vi "Write Response OK.vi"(0 "connection ID":refnum<k5>, 7 "Payload":string="{}", 9 "timeout (ms)":i32=5000, 11 "error in (no error)":errorcluster) -> (4 "connection ID out":refnum<k5>, 15 "error out":errorcluster)   [LabVIEW 2020, in "epl-network.lvlib"]
uses:
  epl-network.lvlib
  Typedefs/TCP Message.ctl
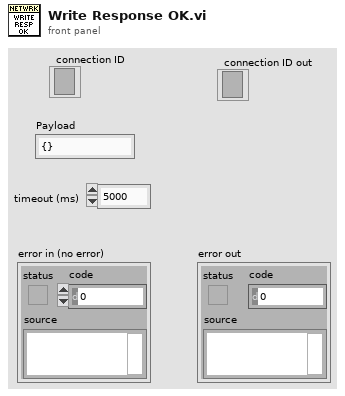
[diagram p1: front panel]
types:
  T1 = typedef "epl-network.lvlib/TCP Message.ctl" = cluster{"Code":i32, "Command":string, "Payload":string}
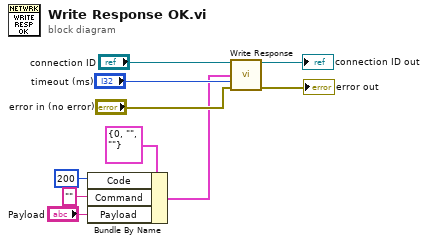
[diagram p0: block diagram]
diagram:
  n1 = Bundle By Name(cluster=T1 {"Code"=0, "Command"="", "Payload"=""} ("TCPMessage"), "Code"=200, "Command"="", "Payload"="Payload") -> (w3:T1)
  n2 = call "Write Response.vi"("connection ID"="connection ID", "TCPMessage"=w3, "timeout (ms)"="timeout (ms)", "error in (no error)"="error in (no error)") -> ("connection ID out"=→"connection ID out":refnum<k5>, "error out"=→"error out":errorcluster)  [unwired: 10 in]
